vi "Config Test.vi"   [LabVIEW 2017]
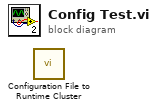
[diagram p0: block diagram]
diagram:
  n1 = call "Configuration File to Runtime Cluster.vi"() -> ()  [unwired: 10 in, 2 out]
